vi "3.1.vi"() -> ()   [LabVIEW 2017]
panel:
  out "数值 4":dbl
  in  "数值 3":dbl
  out "数值 2":dbl
  in  "数值":dbl
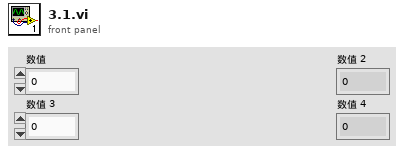
[diagram p1: front panel]
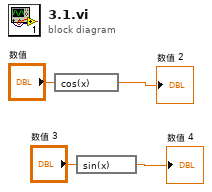
[diagram p0: block diagram]
diagram:
  n1 = expression code="cos(x)"("数值") -> (→"数值 2":dbl)
  n2 = expression code="sin(x)"("数值 3") -> (→"数值 4":dbl)
